vi "Prompt APU Select.vi"(8 "error in (no error)":errorcluster) -> (0 "error out":errorcluster)   [LabVIEW 2018, in "Controller (Host).lvlib"]
doc: "This subVI enqueues the named action in to the communications queue along with the input data."
uses:
  Controller (Host).lvlib
  Private Controls/Module Data.ctl
  Private Controls/Module Action.ctl
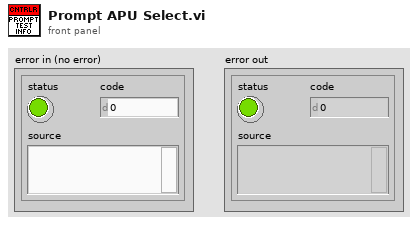
[diagram p1: front panel]
types:
  T1 = typedef "Controller (Host).lvlib/Module Data.ctl" = cluster{"Data":variant, "Action":T2}
  T2 = typedef "Controller (Host).lvlib/Module Action.ctl" = enum8{"Timeout", "New Data", "Value to Monitor", "Init", "Reset Dev_Min_Max", "Error", "Exit", "Prompt Test Info", "Update Test Info", "Prompt Variable Info", "Load APU Setup Data"}
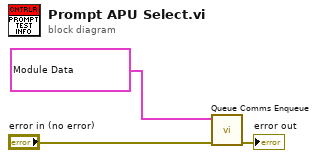
[diagram p0: block diagram]
diagram:
  n1 = call "Queue Comms Enqueue.vi"("error in (no error)"="error in (no error)", "element"=T1 {"Data"=variant, "Action"=enum."Prompt Test Info"} ("Module Data")) -> ("error out"=→"error out":errorcluster)  [unwired: 9 in]
